vi "Drive Controller.vi"(8 "error in":errorcluster) -> ()   [LabVIEW 2025]
doc: "This VI executes continuously carrying out the current operation and responding to updates or new operation requests. It will often contain the timing or control code that is difficult to place directly in TeleOp. This VI generally opens all sensors and motors and isolates the rest of the robot code from knowing implementation details of how the operations are carried out."
uses:
  Drive Setpoints.ctl
  Drive Operations.ctl
  swerve-template/Type Definitions/Data/Robot Velocities.ctl
  <vilib>/Rock Robotics/WPI/ThirdParty/REV Robotics/REVLib/Typedef/Spark MAX Control Type.ctl
  80b923c8-6b82-42f9-a8cd-acddf0fa8107.vi
  Framework/Robot Global Data.vi
panel:
  in  "Drive Controller Diagnostics":T1(tab)
  out "Swerve Visualizer":cluster{dbl[], dbl[]}[](graph)
  out "Pod Comparisons (Diff -> Setpoint - Actual)":T2
  out "(Calibration) Steering Angles":T3
  out "Current\nCmd":string
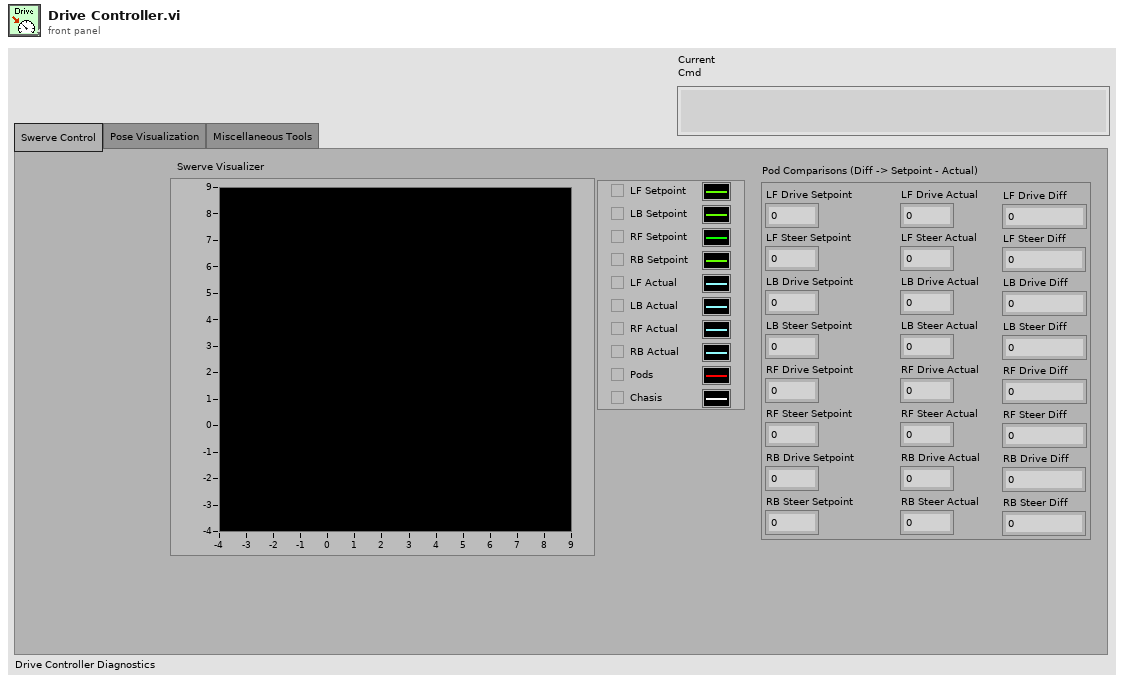
[diagram p1: front panel]
types:
  T1 = enum32{"Swerve Control", "Pose Visualization", "Miscellaneous Tools"}
  T2 = cluster{"LF Drive Setpoint":dbl, "LF Steer Setpoint":dbl, "LB Drive Setpoint":dbl, "LB Steer Setpoint":dbl, "RF Drive Setpoint":dbl, "RF Steer Setpoint":dbl, "RB Drive Setpoint":dbl, "RB Steer Setpoint":dbl, "LF Drive Actual":dbl, "LF Steer Actual":dbl, "LB Drive Actual":dbl, "LB Steer Actual":dbl, "RF Drive Actual":dbl, "RF Steer Actual":dbl, "RB Drive Actual":dbl, "RB Steer Actual":dbl, "LF Drive Diff":dbl, "LF Steer Diff":dbl, "LB Drive Diff":dbl, "LB Steer Diff":dbl, "RF Drive Diff":dbl, "RF Steer Diff":dbl, "RB Drive Diff":dbl, "RB Steer Diff":dbl}
  T3 = cluster{"Left Front":dbl, "Left Back":dbl, "Right Front":dbl, "Right Back":dbl}
  T4 = typedef "Drive Setpoints.ctl" = cluster{"Operation":T5, "Robot Velocities":T6, "Auto Data":cluster{cluster{"Velocities":T6[]}[], cluster{"Positions":cluster{"x":dbl, "y":dbl, "th":dbl}[]}[], cluster{dbl, "Command out":cluster{"Name":string, "vi reference":refnum<vi>, i32[], variant[]}}[], cluster{"Zero Velocity?":bool[]}[], dbl[]}}
  T5 = typedef "Drive Operations.ctl" = enum16{"Reserve", "Read Current", "Immediate", "Calibrate", "Auto", "Auto Pickup"}
  T6 = typedef "Robot Velocities.ctl" = cluster{"X Velocity":dbl, "Y Velocity":dbl, "Rotational \nVelocity":dbl}
  T7 = typedef "(NEO-NEO-ThroughBore-Pigeon2) Swerve.ctl" = cluster{"Drive Motors (NEO)":T8, "Steer Motors (NEO)":T8, "PigeonIMUDevRef":T14, "Radii (ft)":T16}
  T8 = typedef "(NEO & NEO 550) 4 Motor Set.ctl" = cluster{"Left Front":T9, "Left Back":T9, "Right Front":T9, "Right Back":T9}
  T9 = typedef "WPI_MotorControlDeviceRef.ctl" = cluster{"DeviceStatus":errorcluster, "Type":T10, "PWM":cluster{"PWM Channel":T11, "DeadBand":T12}, "CAN":cluster{"Device Number":u8, "SetOutput VI Ref":variant, "GetOutput VI Ref":variant, "Enable VI Ref":variant, "Disable VI Ref":variant, "Data":variant}, "Invert":bool, "DIO PWM":cluster{"PWM \"Enable\" Channel":T11, "DIOChannel":T13, "PWM Rate":dbl}}
  T10 = typedef "WPI_MotorControlType.ctl" = enum16{"PWM", "CAN", "DIO PWM"}
  T11 = typedef "FPGA_DIOPWMChannel.ctl" = enum8{"PWM 0", "PWM 1", "PWM 2", "PWM 3", "PWM 4", "PWM 5", "PWM 6", "PWM 7", "PWM 8", "PWM 9", "PWM MXP 0", "PWM MXP 1", "PWM MXP 2", "PWM MXP 3", "PWM MXP 4", "PWM MXP 5", "PWM MXP 6", "PWM MXP 7", "PWM MXP 8", "PWM MXP 9", "Invalid"}
  T12 = typedef "WPI_PWMDeadband.ctl" = cluster{"Name":string, "maxPositivePwm":i32, "minPositivePwm":i32, "centerPwm":i32, "maxNegativePwm":i32, "minNegativePwm":i32, "angularRange":u16}
  T13 = typedef "FPGA_DIOChannel.ctl" = enum8{"DIO 0", "DIO 1", "DIO 2", "DIO 3", "DIO 4", "DIO 5", "DIO 6", "DIO 7", "DIO 8", "DIO 9", "DIO MXP 0", "DIO MXP 1", "DIO MXP 2", "DIO MXP 3", "DIO MXP 4", "DIO MXP 5", "DIO MXP 6", "DIO MXP 7", "DIO MXP 8", "DIO MXP 9", "DIO MXP 10", "DIO MXP 11", "DIO MXP 12", "DIO MXP 13", "DIO MXP 14", "DIO MXP 15", "SPI Port CS1", "SPI Port CS2", "SPI Port CS3", "SPI Port MISO", "SPI Port MOSI", "Invalid"}
  T14 = typedef "CTRE_PigeonIMU_DeviceRef.ctl" = cluster{"DeviceStatus":errorcluster, "Device Number":u8, "Type":T15, "Device ID":u32, "Handle":u64, "UsageFrame":u32, "Library Path":path}
  T15 = typedef "CTRE_PigeonIMU_ConnectionType.ctl" = u32
  T16 = typedef "Pod Positions.ctl" = cluster{"Left Front Position":dbl[], "Left Back Position":dbl[], "Right Front Position":dbl[], "Right Back Position":dbl[]}
  T17 = typedef "Command Status Info.ctl" = cluster{"Name":string, "Status":T18, "notifier out":T19}
  T18 = typedef "Completion Status.ctl" = enum16{"Successful", "Aborted", "Incomplete"}
  T19 = typedef "Completion Notifier.ctl" = refnum<notifier>
  T20 = cluster{"SubSystem Data":T4, cluster{"Start Time (ms)":u32, "Iterations":i32}, cluster{"Command Info":T17, "Description":string, "Default Command":T4, "queue out":refnum<queue>, "Subsystem Name":string}}
  T21 = cluster{"Auto Velocities":T6[], "Auto Positions":cluster{"x":dbl, "y":dbl, "th":dbl}[], "Auto Commands":cluster{dbl, "Command out":cluster{"Name":string, "vi reference":refnum<vi>, i32[], variant[]}}[], "Zero Velocity?":bool[]}
  T22 = cluster{cluster{"Velocities":T6[]}[], cluster{"Positions":cluster{"x":dbl, "y":dbl, "th":dbl}[]}[], cluster{dbl, "Command out":cluster{"Name":string, "vi reference":refnum<vi>, i32[], variant[]}}[], cluster{"Zero Velocity?":bool[]}[], dbl[]}
  T23 = typedef "Drive Conditions.ctl" = cluster{"Field Centric":bool, "BotPose Correction":bool, "Theta Align":bool, "Current Limit 50A(F) 60A(T)":bool, "Align to Bump or Shoot":bool}
  T24 = typedef "Spark MAX Control Type.ctl" = enum16{"Percent VBus", "Voltage", "Velocity", "Position", "Smart Motion", "Current", "Smart Velocity", "MAXMotion Position", "MAXMotion Velocity"}
  T25 = cluster{"SubSystem Data":T4, cluster{"Start Time (ms)":u32, "Iterations":i32}, "Default Command Arguments":cluster{"Command Info":T17, "Description":string, "Default Command":T4, "queue out":refnum<queue>, "Subsystem Name":string}}
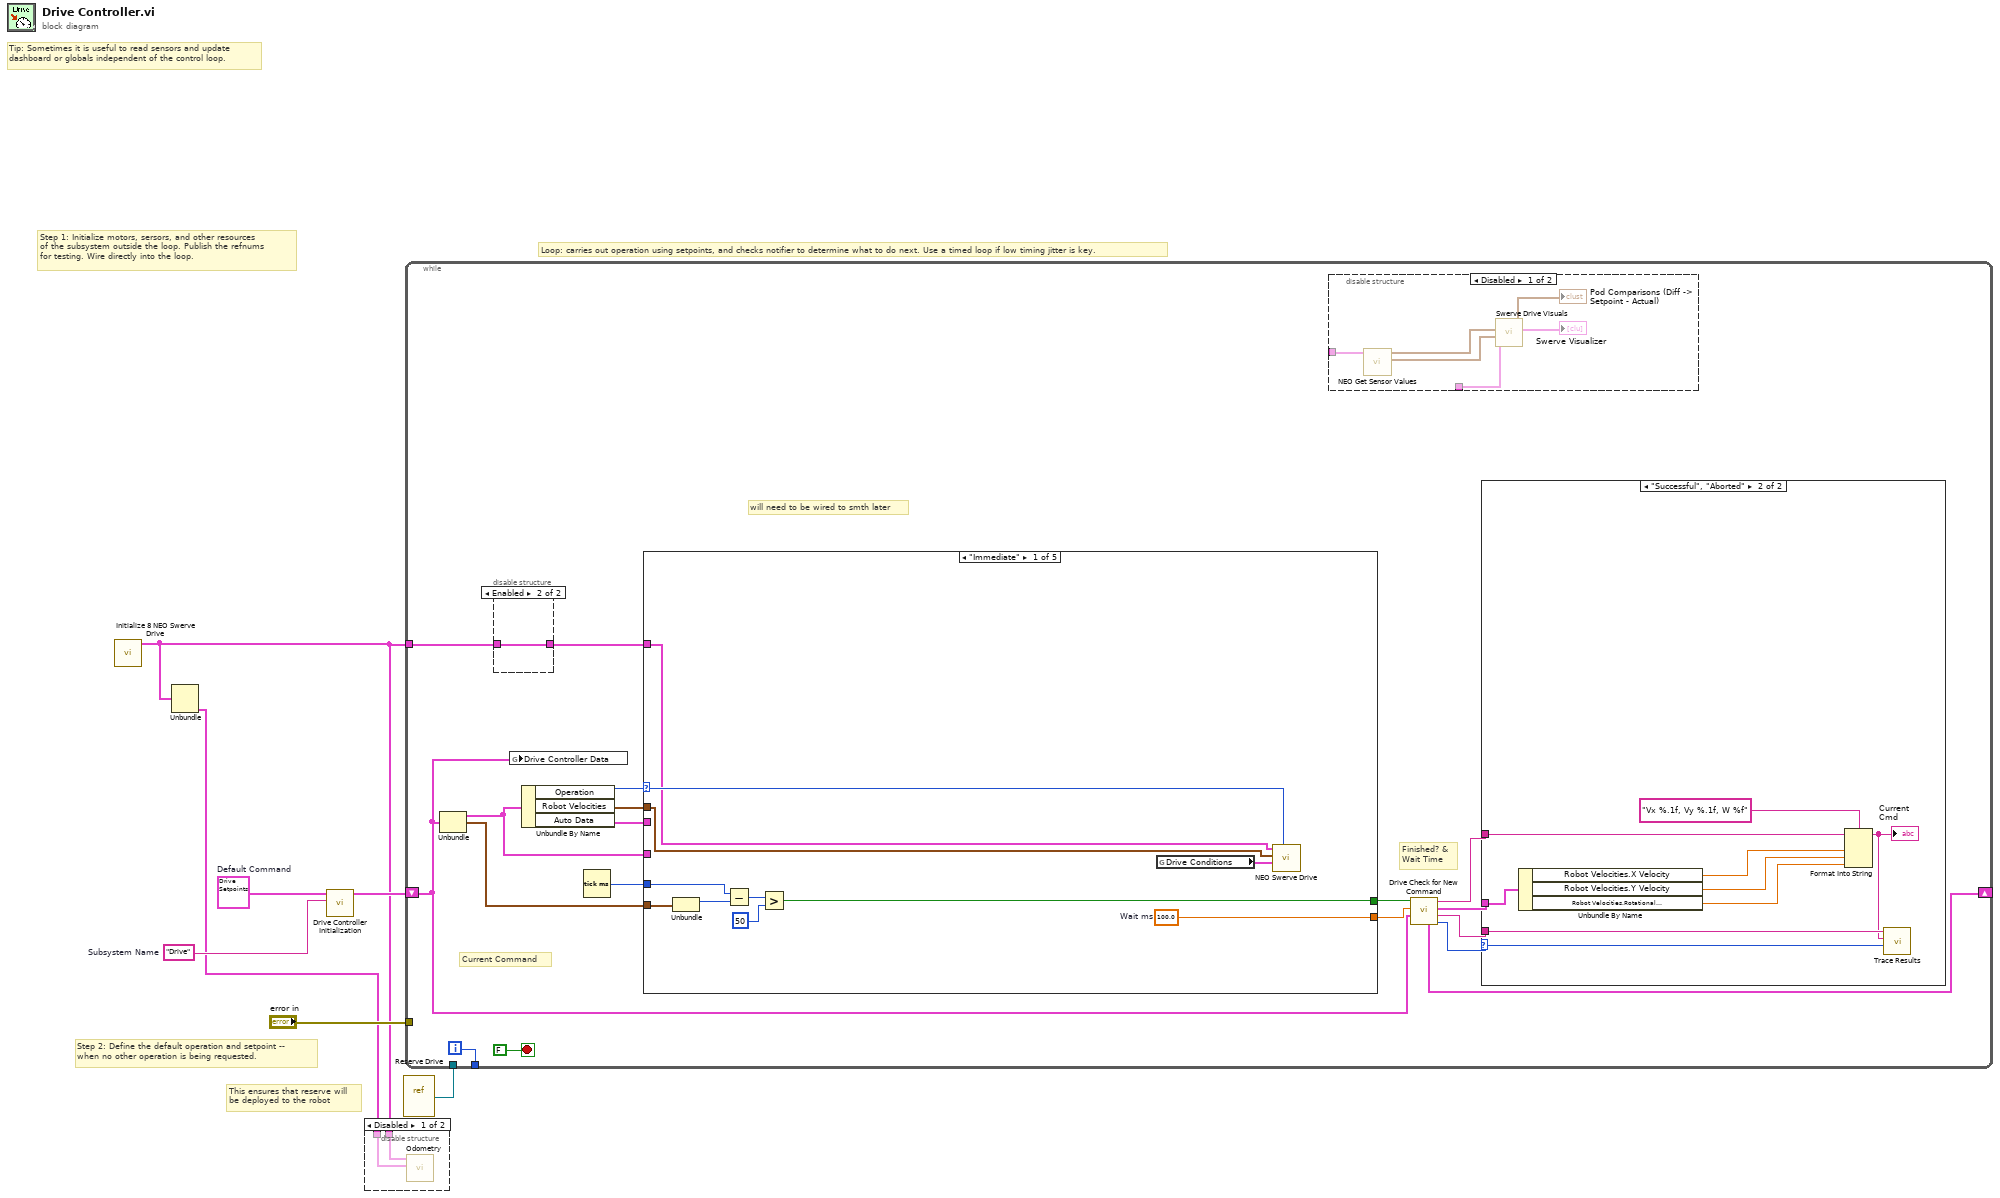
[diagram p0: block diagram]
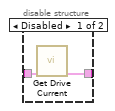
[diagram p3: hidden frame]
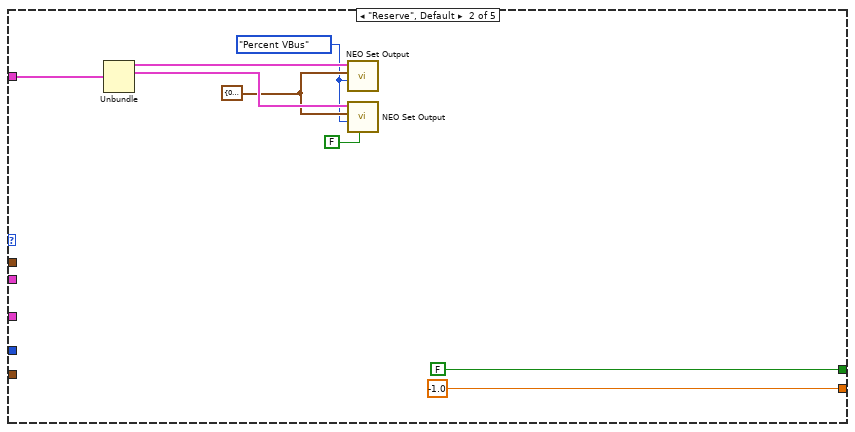
[diagram p5: hidden frame]
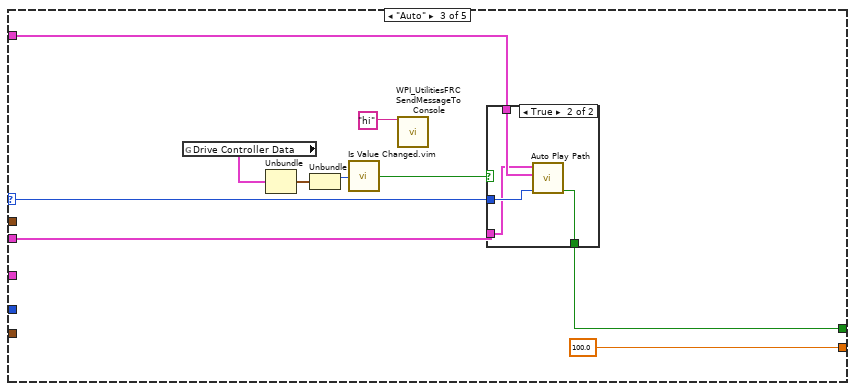
[diagram p6: hidden frame]
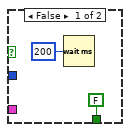
[diagram p7: hidden frame]
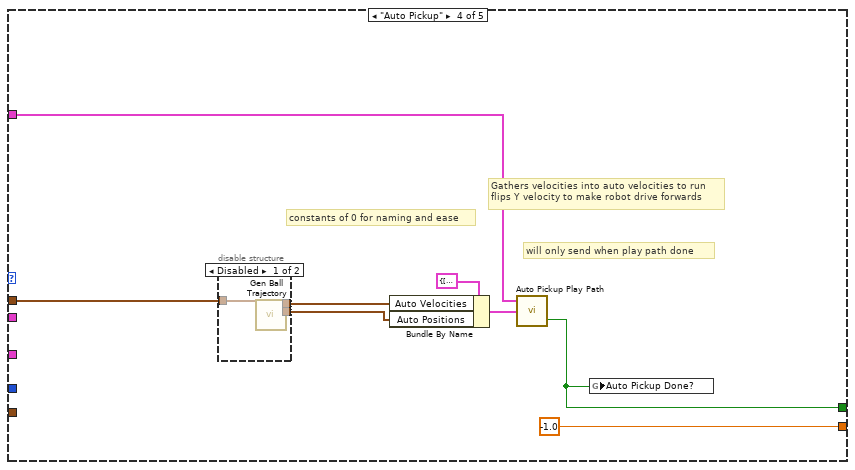
[diagram p8: hidden frame]
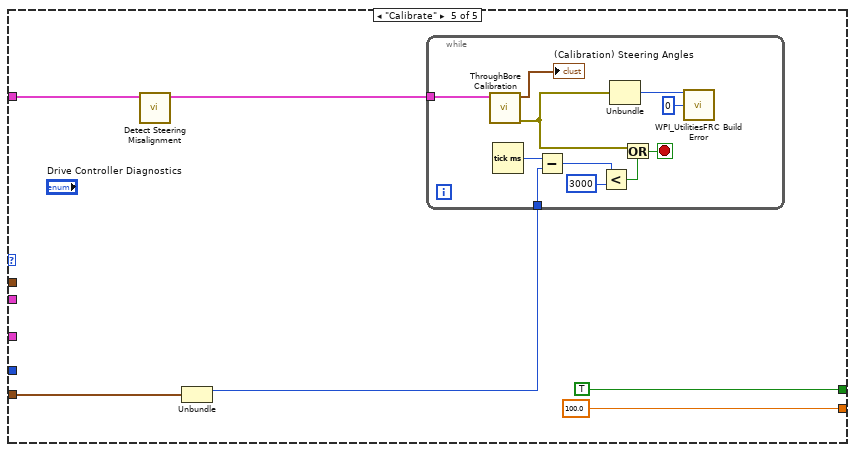
[diagram p10: hidden frame]
diagram:
  w3 = T4 {"Operation"=enum."Reserve", "Robot Velocities"={"X Velocity"=0.0, "Y Velocity"=0.0, "Rotational \nVelocity"=0.0}, "Auto Data"={[], [], [], [], []}}  # Default Command
  w7 = "Drive"  # Subsystem Name
  # "This ensures that reserve will\nbe deployed to the robot"
  # "Step 2: Define the default operation and setpoint --\nwhen no other operation is being requested."
  # "Step 1: Initialize motors, sersors, and other resources\nof the subsystem outside the loop. Publish the refnums\nfor testing. Wire directly into the loop."
  # "Loop: carries out operation using setpoints, and checks notifier to determine what to do next. Use a timed loop if low timing jitter is key."
  # "Tip: Sometimes it is useful to read sensors and update\ndashboard or globals independent of the control loop."
  n1 = call "Initialize 8 NEO Swerve Drive.vi"() -> ("Motors"=w1:T7)  [unwired: 10 in, 1 out]
  n2 = Unbundle(w1) -> ("Radii (ft)"=w2:T16)  [unwired: 3 out]
  n3 = call "Drive Controller Initialization.vi"("Subsystem Name"=w7, "Default Command"=w3) -> ("Current Command"=w5:T20)  [unwired: 9 in]
  n4 = disable-structure shown="Disabled" {
    disable-tunnel: w2 -> [w9 _]
    disable-tunnel: w1 -> [w8 _]
    frame Disabled {
      n5 = call "Odometry.vi"("Radii (ft)"=w9, "Motors"=w8) -> ()  [unwired: 10 in]
    }
    frame Enabled {
    }
  }
  n6 = vi-ref "Reserve Drive.vi"() -> (w4:refnum<vi>)
  n7 = while {
    shift-right: [w20] -> _
    shift-left: w5 -> [w12]
    tunnel: [w26] -> _
    tunnel: "error in" -> [_]
    tunnel: w4 -> [_]
    tunnel: w1 -> [w11]
    i -> [w26]
    stop <- FALSE stop-if-true
    # "will need to be wired to smth later"
    # "Current Command"
    # "Finished? &\nWait Time"
    n8 = Unbundle(w12) -> ("SubSystem Data"=w15:T4, w13:cluster{"Start Time (ms)":u32, "Iterations":i32})  [unwired: 1 out]
    n9 = disable-structure shown="Enabled" {
      disable-tunnel: w11 -> [w29 w30]
      disable-tunnel: [w28 w30] -> w10
      frame Disabled {
        n10 = call "Get Drive Current.vi"("Motors In"=w29) -> ("Motors Out"=w28:T7)  [unwired: 10 in]
      }
      frame Enabled {
      }
    }
    n11 = global write "Robot Global Data.vi" "Drive Controller Data"(w12) -> ()
    n12 = Unbundle By Name(w15) -> ("Operation"=w18:T5, "Robot Velocities"=w21:T6, "Auto Data"=w19:T22)
    n13 = Tick Count (ms)() -> (millisecond timer value=w14:u32)
    n14 = case shown="\"Immediate\"" w18 {
      selector: w18 -> [w39 _ w59 _ _]
      tunnel: [w47 -1.0 ("Infinite") 100.0 -1.0 ("Infinite") 100.0 ("Infinite")] -> w25
      tunnel: [w42 FALSE ("ignore previous (F)") w58 w74 TRUE ("ignore previous (F)")] -> w24
      tunnel: w13 -> [w46 _ _ _ w86]
      tunnel: w14 -> [w41 _ _ _ _]
      tunnel: w21 -> [w37 _ _ w79 _]
      tunnel: w10 -> [w38 w53 w65 w78 w84]
      tunnel: w15 -> [_ _ _ _ _]
      tunnel: w19 -> [_ _ w57 _ _]
      frame "Immediate" {
        w47 = 100.0  # Wait ms
        n15 = Unbundle(w46) -> ("Start Time (ms)"=w45:u32)  [unwired: 1 out]
        n16 = Subtract(x=w41, y=w45) -> (x-y=w44:u32)
        n17 = Greater?(x=w44, y=u32 50) -> (0:w42:bool)
        n18 = global read "Robot Global Data.vi" "Drive Conditions"() -> (w40:T23)
        n19 = call "NEO Swerve Drive.vi"("Operation"=w39, "Drive Conditions"=w40, "Robot Velocities"=w37, "Swerve Drive"=w38) -> ()  [unwired: 6 in, 2 out]
      }
      frame "Reserve", Default {
        w48 = Spark_MAX_Control_Type."Percent VBus" ("Reserve Control Mode")
        w49 = T3 {"Left Front"=0.0, "Left Back"=0.0, "Right Front"=0.0, "Right Back"=0.0} ("Setpoints")
        n20 = Unbundle(w53) -> ("Drive Motors (NEO)"=w52:T8, "Steer Motors (NEO)"=w51:T8)  [unwired: 2 out]
        n21 = call "NEO Set Output.vi"("Control Mode"=w48, "Setpoints"=w49, "Motors"=w52) -> ()  [unwired: 9 in]
        n22 = call "NEO Set Output.vi"("Add Angle Offsets?"=FALSE, "Control Mode"=w48, "Setpoints"=w49, "Motors"=w51) -> ()  [unwired: 8 in]
      }
      frame "Auto" {
        n23 = global read "Robot Global Data.vi" "Drive Controller Data"() -> (w63:T20)
        n24 = Unbundle(w63) -> (w62:cluster{"Start Time (ms)":u32, "Iterations":i32})  [unwired: 2 out]
        n25 = Unbundle(w62) -> ("Start Time (ms)"=w61:u32)  [unwired: 1 out]
        n26 = call "Is Value Changed.vim"("value"=w61) -> ("changed or first call?"=w60:bool)
        n27 = call <vilib>:"WPI_UtilitiesFRC SendMessageToConsole.vi"("Message"="hi") -> ()  [unwired: 14 in, 1 out]
        n28 = case shown="True" w60 {
          tunnel: w57 -> [_ w68]
          tunnel: w65 -> [_ w71]
          tunnel: w59 -> [_ w70]
          tunnel: [FALSE ("Auto Done?") w69] -> w58
          frame False {
            n29 = Wait (ms)(milliseconds to wait=u32 200) -> ()  [unwired: 1 out]
          }
          frame True {
            n30 = call "Auto Play Path.vi"("Operation"=w70, "Motors"=w71, "Auto Data"=w68) -> ("Auto Done?"=w69:bool)  [unwired: 6 in, 2 out]
          }
        }
      }
      frame "Auto Pickup" {
        # "will only send when play path done"
        # "constants of 0 for naming and ease"
        # "Gathers velocities into auto velocities to run\nflips Y velocity to make robot drive forwards"
        n31 = disable-structure shown="Disabled" {
          disable-tunnel: w79 -> [w82 _]
          disable-tunnel: [w81 _] -> w73
          disable-tunnel: [w80 _] -> w72
          frame Disabled {
            n32 = call "Gen Ball Trajectory.vi"("Robot Velocities"=w82) -> ("Auto Positions"=w80:cluster{"x":dbl, "y":dbl, dbl}[], "Auto Velocities"=w81:cluster{"x out":dbl, "y out":dbl, "Omega":dbl}[])  [unwired: 9 in]
          }
          frame Enabled {
          }
        }
        n33 = Bundle By Name(cluster=T21 {"Auto Velocities"=[], "Auto Positions"=[], "Auto Commands"=[], "Zero Velocity?"=[]} ("Auto Data"), "Auto Velocities"=w73, "Auto Positions"=w72) -> (w75:T21)
        n34 = call "Auto Pickup Play Path.vi"("Auto Data"=w75, "Motors"=w78) -> ("Align Good?"=w74:bool)  [unwired: 2 in]
        n35 = global write "Robot Global Data.vi" "Auto Pickup Done?"(w74) -> ()
      }
      frame "Calibrate" {
        n36 = call "Detect Steering Misalignment.vi"("Motors In"=w84) -> ("Motors Out"=w83:T7)  [unwired: 10 in]
        n37 = Unbundle(w86) -> ("Start Time (ms)"=w85:u32)  [unwired: 1 out]
        n38 = while {
          tunnel: w83 -> [w93]
          tunnel: w85 -> [w98]
          stop <- w99 stop-if-true
          n39 = call "ThroughBore Calibration.vi"("Motors"=w93) -> ("error out"=w90:errorcluster, "Steering Angles"=→"(Calibration) Steering Angles":cluster{"LF":dbl, "LB":dbl, "RF":dbl, "RB":dbl})  [unwired: 9 in]
          n40 = Tick Count (ms)() -> (millisecond timer value=w97:u32)
          n41 = Subtract(x=w97, y=w98) -> (x-y=w96:u32)
          n42 = Less?(x=w96, y=u32 3000) -> (x < y?=w94:bool)
          n43 = Unbundle(w90) -> ("code"=w89:i32)  [unwired: 2 out]
          n44 = Or(x=w90, y=w94) -> (x .or. y?=w99:bool)
          n45 = call <vilib>:"WPI_UtilitiesFRC Build Error.vi"("error code"=w89, "chain levels to remove (1)"=0) -> ()  [unwired: 3 in, 11 out]
        }
      }
    }
    n46 = disable-structure shown="Disabled" {
      disable-tunnel: _ -> [w34 _]
      disable-tunnel: _ -> [w31 _]
      frame Disabled {
        n47 = call "NEO Get Sensor Values.vi"("Swerve Motors"=w31) -> ("Steer Angles (degrees)"=w32:T3, "Drive Velocities (ft/s)"=w33:T3)  [unwired: 9 in]
        n48 = call "Swerve Drive Visuals.vi"("Steer Angles (degrees)"=w32, "Drive Velocities (ft/s)"=w33, "Pod Setpoints (ft/s and deg)"=w34) -> ("Swerve Visualizer"=→"Swerve Visualizer":cluster{dbl[], dbl[]}[], "Pod Comparisons (Diff -> Setpoint - Actual)"=→"Pod Comparisons (Diff -> Setpoint - Actual)":T2)  [unwired: 7 in]
      }
      frame Enabled {
      }
    }
    n49 = call "Drive Check for New Command.vi"("input cluster"=w12, "Wait time (ms)"=w25, "Finished?"=w24) -> ("Completion"=w17:T18, "Subsystem Name"=w22:string, "Current Command"=w16:T4, "Initial Trace String"=w23:string, "Next Command"=w20:T25)  [unwired: 4 in]
    n50 = case shown="\"Successful\", \"Aborted\"" w17 {
      selector: w17 -> [_ w100]
      tunnel: w23 -> [_ w107]
      tunnel: w16 -> [_ w108]
      tunnel: w22 -> [_ w106]
      frame "Incomplete", Default {
        # "Continuing current command"
      }
      frame "Successful", "Aborted" {
        # "Report and setup for next command"
        n51 = Unbundle By Name(w108) -> ("Robot Velocities.X Velocity"=w104:dbl, "Robot Velocities.Y Velocity"=w105:dbl, "Robot Velocities.Rotational \nVelocity"=w101:dbl)
        n52 = Format Into String(format string="Vx %.1f, Vy %.1f, W %f", initial string=w107, w104, w105, w101) -> (resulting string=w102:string)  [unwired: 1 in, 1 out]
        "Current\nCmd" <- w102
        n53 = call <vilib>:"Trace Results.vi"("Status of previous command"=w100, "Description"=w102, "Subsystem"=w106) -> ()  [unwired: 9 in]
      }
    }
  }
